vi "Read All FP Properties.vi"(8 "error in (no error)":errorcluster, 9 "No Error clusters":bool, 10 "Is On Connector Pane":bool, 11 "VI in":refnum<vi>) -> (0 "error out":errorcluster, 2 "Outputs":T1, 3 "Inputs":T1)   [LabVIEW 2020, in "DocTool.lvlib"]
uses:
  DocTool.lvlib
  TDefs/FP Items Properties.ctl
  TDefs/FP Item Properties.ctl
  TDefs/CopyTag.ctl
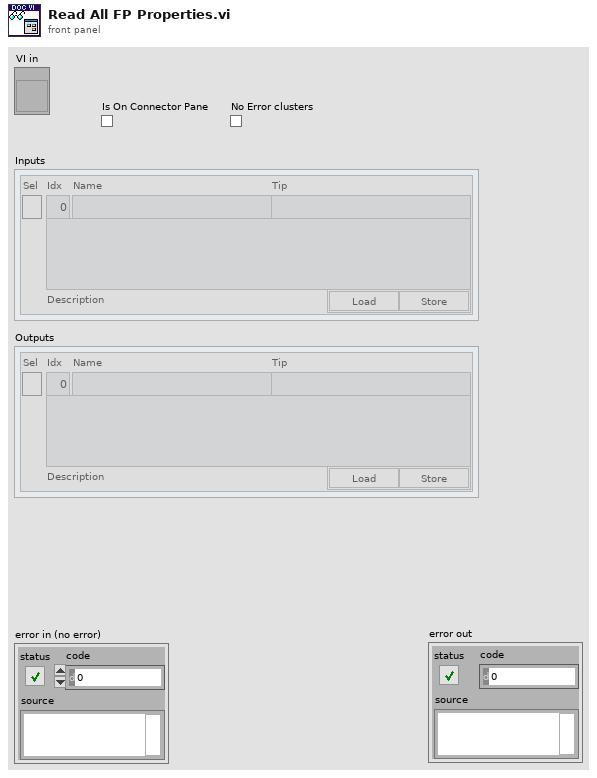
[diagram p1: front panel]
types:
  T1 = typedef "DocTool.lvlib/FP Items Properties.ctl" = T2[]
  T2 = typedef "DocTool.lvlib/FP Item Properties.ctl" = cluster{"Sel":bool, "Idx":i32, "Name":string, "Description":string, "Tip":string, "Load Store":T3}
  T3 = typedef "DocTool.lvlib/CopyTag.ctl" = cluster{"Load":bool, "Store":bool}
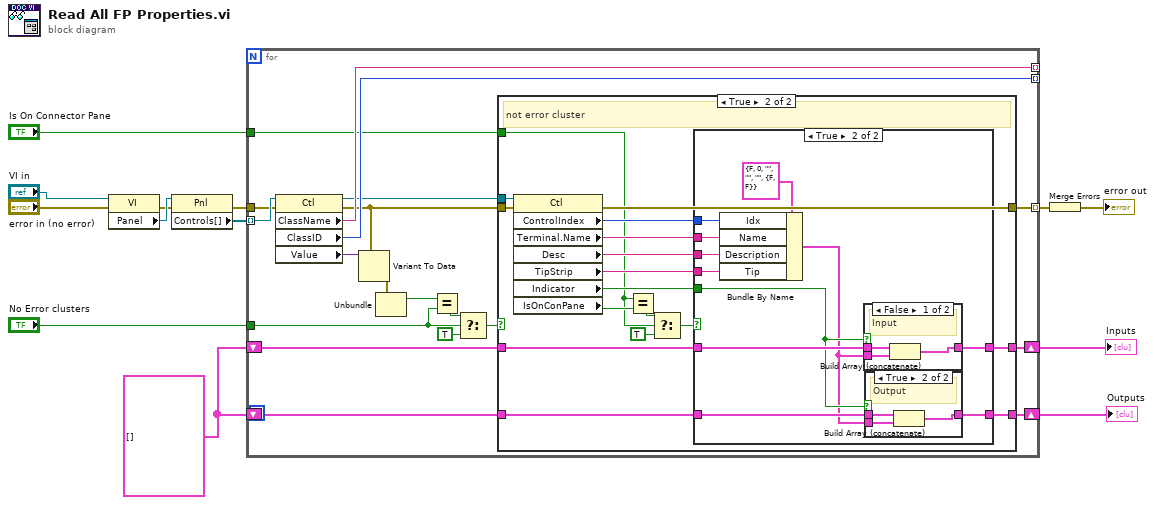
[diagram p0: block diagram]
diagram:
  w4 = T1 [] ("FP Items")
  n1 = property class="VI"(reference="VI in", error in="error in (no error)") -> (error out=w7:errorcluster, "Panel"=w10:refnum<vi>)  [unwired: 1 out]
  n2 = property class="Pnl"(reference=w10, error in=w7) -> (error out=w8:errorcluster, "Controls[]"=w9:refnum<vi>[])  [unwired: 1 out]
  n3 = for {
    tunnel: w9 -> [w32] mode=indexing
    tunnel: [w30] -> _ mode=indexing
    tunnel: [w31] -> _ mode=indexing
    tunnel: w8 -> [w28]
    tunnel: [w27] -> w11 mode=indexing
    shift-right: [w23] -> w5
    shift-left: w4 -> [w24]
    shift-right: [w25] -> w3
    shift-left: w4 -> [w26]
    tunnel: "Is On Connector Pane" -> [w22]
    tunnel: "No Error clusters" -> [w16]
    n4 = property class="Ctl"(reference=w32, error in=w28) -> (reference out=w29:refnum<vi>, error out=w20:errorcluster, "ClassName"=w30:string, "ClassID"=w31:u32, "Value"=w21:variant)
    n5 = Variant To Data(type=w20, Variant=w21) -> (error out=w19:errorcluster)  [unwired: 1 in, 1 out]
    n6 = Unbundle(w19) -> ("status"=w15:bool)  [unwired: 2 out]
    n7 = Equal?(x=w15, y=w16) -> (x = y?=w18:bool)
    n8 = Select(t=w18, s=w16, f=TRUE) -> (s? t:f=w14:bool)
    n9 = case shown="True" w14 {
      tunnel: w29 -> [_ w52]
      tunnel: [w35 w51] -> w27
      tunnel: w26 -> [w33 w50]
      tunnel: [w33 w49] -> w25
      tunnel: w24 -> [w34 w44]
      tunnel: [w34 w42] -> w23
      tunnel: w22 -> [_ w40]
      tunnel: w20 -> [w35 w36]
      frame False {
      }
      frame True {
        # "not error cluster"
        n10 = property class="Ctl"(reference=w52, error in=w36) -> (error out=w51:errorcluster, "ControlIndex"=w45:i32, "Terminal.Name"=w46:string, "Desc"=w47:string, "TipStrip"=w48:string, "Indicator"=w43:bool, "IsOnConPane"=w41:bool)  [unwired: 1 out]
        n11 = Equal?(x=w40, y=w41) -> (x = y?=w39:bool)
        n12 = Select(t=w39, s=w40, f=TRUE) -> (s? t:f=w37:bool)
        n13 = case shown="True" w37 {
          tunnel: w50 -> [w53 w65]
          tunnel: [w53 w64] -> w49
          tunnel: w48 -> [_ w62]
          tunnel: w47 -> [_ w61]
          tunnel: w46 -> [_ w60]
          tunnel: w45 -> [_ w59]
          tunnel: w44 -> [w54 w58]
          tunnel: w43 -> [_ w57]
          tunnel: [w54 w55] -> w42
          frame False {
          }
          frame True {
            n14 = Bundle By Name(cluster=T2 {"Sel"=FALSE, "Idx"=0, "Name"="", "Description"="", "Tip"="", "Load Store"={"Load"=FALSE, "Store"=FALSE}} ("FP Item Properties"), "Idx"=w59, "Name"=w60, "Description"=w61, "Tip"=w62) -> (w56:T2)
            n15 = case shown="False" w57 {
              tunnel: w58 -> [w68 w69]
              tunnel: [w67 w69] -> w55
              tunnel: w56 -> [w66 _]
              frame False {
                # "Input"
                n16 = Build Array (concatenate)(w68, w66) -> (w67:T1)
              }
              frame True {
              }
            }
            n17 = case shown="True" w57 {
              tunnel: w65 -> [w70 w73]
              tunnel: [w70 w72] -> w64
              tunnel: w56 -> [_ w71]
              frame False {
              }
              frame True {
                # "Output"
                n18 = Build Array (concatenate)(w73, w71) -> (w72:T1)
              }
            }
          }
        }
      }
    }
  }
  "Inputs" <- w5
  "Outputs" <- w3
  n19 = Merge Errors(w11) -> (→"error out":errorcluster)
